vi "DrawToXYgraph.vi"(6 "BaseTimeCluster":refnum<vi>, 9 "XYGraphData":refnum<vi>, 10 "TimeFormat":refnum<vi>, 11 "XYGraph输入":refnum<vi>) -> ()   [LabVIEW 2015]
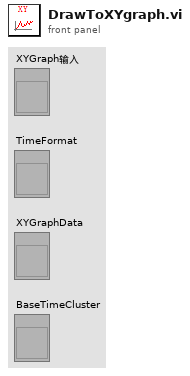
[diagram p1: front panel]
types:
  T1 = cluster{"基时间字符串":string, "基时间秒":dbl, "基时间标识":timestamp}
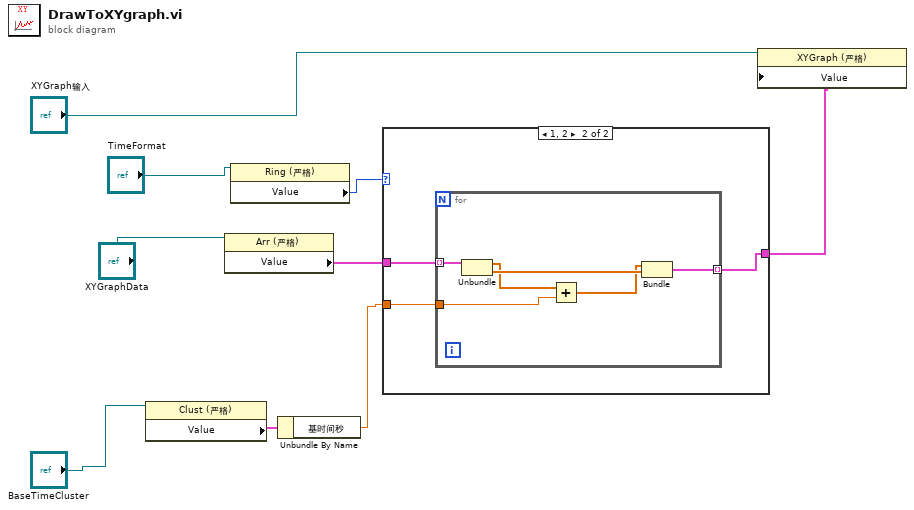
[diagram p0: block diagram]
diagram:
  n1 = property class="Clust (严格)"(reference="BaseTimeCluster") -> ("Value"=w8:T1)  [unwired: 1 in, 2 out]
  n2 = property class="Arr (严格)"(reference="XYGraphData") -> ("Value"=w5:cluster{"时间(s)":dbl[], "数据":dbl[]}[])  [unwired: 1 in, 2 out]
  n3 = property class="Ring (严格)"(reference="TimeFormat") -> ("Value"=w4:u16)  [unwired: 1 in, 2 out]
  n4 = Unbundle By Name(w8) -> ("基时间秒"=w9:dbl)
  n5 = case shown="1, 2" w4 {
    tunnel: [w10 w12] -> w6
    tunnel: w5 -> [w10 w13]
    tunnel: w9 -> [_ w11]
    frame 0, Default {
    }
    frame 1, 2 {
      n6 = for {
        tunnel: w13 -> [w19] mode=indexing
        tunnel: [w18] -> w12 mode=indexing
        tunnel: w11 -> [w16]
        n7 = Unbundle(w19) -> ("时间(s)"=w15:dbl[], "数据"=w17:dbl[])
        n8 = Add(x=w15, y=w16) -> (x+y=w14:dbl[])
        n9 = Bundle(w14, "数据"=w17) -> (w18:cluster{dbl[], "数据":dbl[]})  [unwired: 1 in]
      }
    }
  }
  n10 = property class="XYGraph (严格)"(reference="XYGraph输入", "Value"=w6) -> ()  [unwired: 1 in, 2 out]
